vi "Write ID.vi"(8 "error in (no error)":errorcluster, 10 "ID":i32, 11 "Philosopher in":refnum<class "Philosopher.lvclass">) -> (0 "error out":errorcluster, 3 "Philosopher out":refnum<class "Philosopher.lvclass">)   [LabVIEW 2023, in "Philosopher.lvlib" / "Philosopher.lvclass"]
uses:
  Philosopher.lvclass
  Philosopher.lvclass/Philosopher.ctl
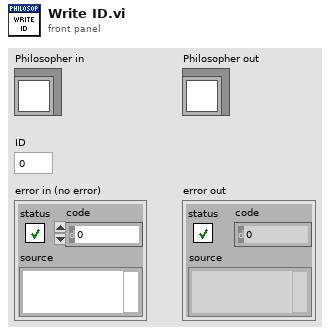
[diagram p1: front panel]
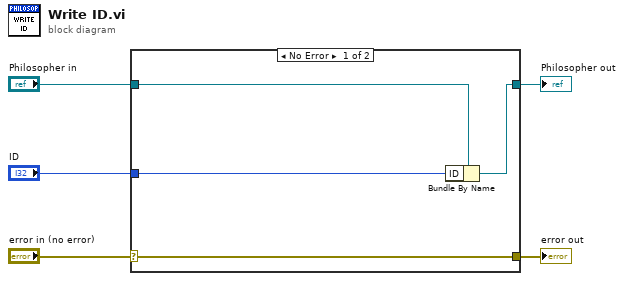
[diagram p0: block diagram]
diagram:
  n1 = case shown="No Error" "error in (no error)" {
    selector: "error in (no error)" -> [w9 w10]
    tunnel: [w9 w10] -> w4
    tunnel: [w7 w11] -> w2
    tunnel: "Philosopher in" -> [w8 w11]
    tunnel: "ID" -> [w6 _]
    frame No Error {
      n2 = Bundle By Name(cluster=w8, "ID"=w6) -> (w7:refnum<class "Philosopher.lvclass">)
    }
    frame Error {
    }
  }
  "error out" <- w4
  "Philosopher out" <- w2
